vi "Log Warnings.vi"(8 "Error In":errorcluster, 10 "Weather Data In":T1, 11 "file ref in":refnum<file>) -> (0 "Error Out":errorcluster, 3 "file ref out":refnum<file>)   [LabVIEW 2020]
uses:
  Weather Data.ctl
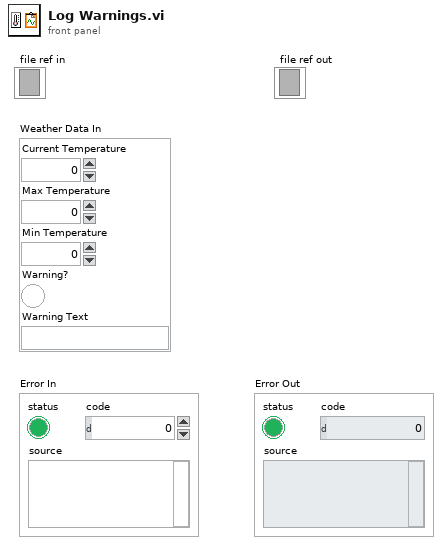
[diagram p1: front panel]
types:
  T1 = typedef "Weather Data.ctl" = cluster{"Current Temperature":dbl, "Max Temperature":dbl, "Min Temperature":dbl, "Warning?":bool, "Warning Text":string}
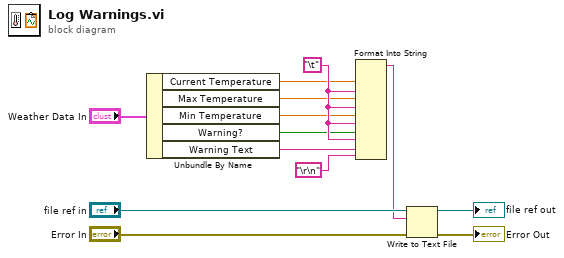
[diagram p0: block diagram]
diagram:
  w13 = "\t"
  n1 = Unbundle By Name("Weather Data In") -> ("Current Temperature"=w11:dbl, "Max Temperature"=w10:dbl, "Min Temperature"=w9:dbl, "Warning?"=w8:bool, "Warning Text"=w7:string)
  n2 = Format Into String(w11, w13, w10, w13, w9, w13, w8, w13, w7, "\r\n") -> (resulting string=w4:string)  [unwired: 3 in, 1 out]
  n3 = Write to Text File(file (use dialog)="file ref in", text=w4, error in="Error In") -> (refnum out=→"file ref out":refnum<file>, error out=→"Error Out":errorcluster)  [unwired: 1 in, 1 out]
